vi "Gen Array.vi"(7 "Steps":i32=1001, 10 "End":dbl=0.5, 11 "Start":dbl=-0.5) -> (3 "Array":dbl[](array[numeric]))   [LabVIEW 2023]
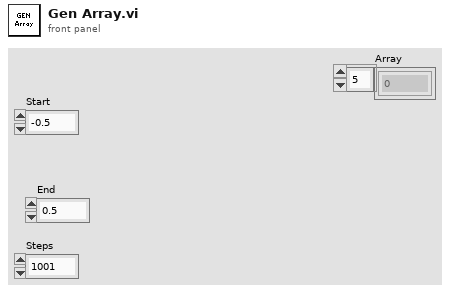
[diagram p1: front panel]
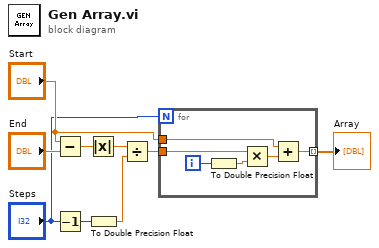
[diagram p0: block diagram]
diagram:
  n1 = Subtract(x="Start", y="End") -> (x-y=w7:dbl)
  n2 = Decrement(x="Steps") -> (x-1=w5:i32)
  n3 = Absolute Value(x=w7) -> (abs(x)=w2:dbl)
  n4 = To Double Precision Float(number=w5) -> (double precision float=w1:dbl)
  n5 = Divide(x=w2, y=w1) -> (x/y=w4:dbl)
  n6 = for {
    N: "Steps" -> [_]
    tunnel: "Start" -> [w15]
    tunnel: w4 -> [w14]
    tunnel: [w10] -> w3 mode=indexing
    i -> [w13]
    n7 = To Double Precision Float(number=w13) -> (double precision float=w12:dbl)
    n8 = Multiply(x=w14, y=w12) -> (x*y=w11:dbl)
    n9 = Add(x=w15, y=w11) -> (x+y=w10:dbl)
  }
  "Array" <- w3
